vi "Create Mask.vi"(4 "Color":u32(colorbox), 6 "Transparency":u8, 8 "Error in":errorcluster caption="Error in (no error)", 10 "Bounds":T1, 11 "Rectangle Mask In":refnum<class "Rectangle Mask.lvclass">) -> (0 "Error out":errorcluster, 3 "Rectangle Mask Out":refnum<class "Rectangle Mask.lvclass">)   [LabVIEW 2016, in "Rectangle Mask.lvclass"]
uses:
  Rectangle Mask.lvclass
  <vilib>/Utility/miscctls.llb/LVRectTypeDef.ctl
  Rectangle Mask.lvclass/Rectangle Mask.ctl
panel:
  in  "Visible":bool
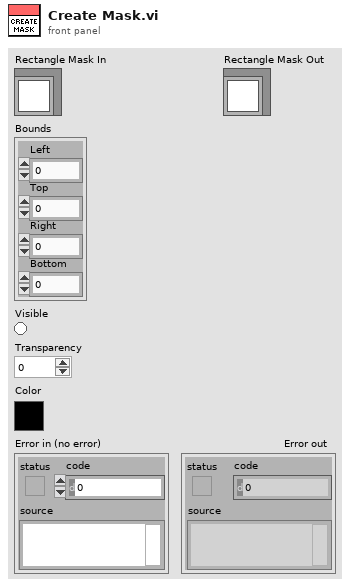
[diagram p1: front panel]
types:
  T1 = typedef "LVRectTypeDef.ctl" = cluster{"Left":i16, "Top":i16, "Right":i16, "Bottom":i16}
  T2 = typedef "Rectangle Mask.lvclass/Panels.ctl" = cluster{"Left":refnum<vi>, "Top":refnum<vi>, "Right":refnum<vi>, "Bottom":refnum<vi>}
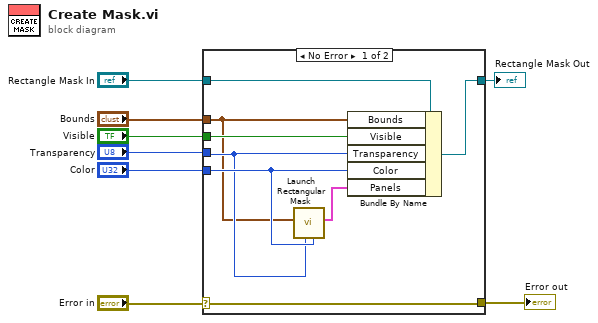
[diagram p0: block diagram]
diagram:
  n1 = case shown="No Error" "Error in" {
    selector: "Error in" -> [w16 w18]
    tunnel: [w16 w18] -> w7
    tunnel: "Rectangle Mask In" -> [w15 w17]
    tunnel: "Bounds" -> [w10 _]
    tunnel: "Visible" -> [w14 _]
    tunnel: "Transparency" -> [w11 _]
    tunnel: "Color" -> [w12 _]
    tunnel: [w13 w17] -> w1
    frame No Error {
      n2 = call "Launch Rectangular Mask.vi"("Color"=w12, "Transparency"=w11, "Bounds"=w10) -> ("Panels (cluster)"=w9:T2)  [unwired: 7 in, 1 out]
      n3 = Bundle By Name(cluster=w15, "Bounds"=w10, "Visible"=w14, "Transparency"=w11, "Color"=w12, "Panels"=w9) -> (w13:refnum<class "Rectangle Mask.lvclass">)
    }
    frame Error {
    }
  }
  "Error out" <- w7
  "Rectangle Mask Out" <- w1
